vi "GetMeasured.vi"(8 "error in (no error)":errorcluster, 11 "CodeCoverage in":refnum<class "CodeCoverage.lvclass">) -> (0 "error out":errorcluster, 2 "All VIs Measured":path[](array[path]), 3 "CodeCoverage out":refnum<class "CodeCoverage.lvclass">)   [LabVIEW 2019, in "CodeCoverage.lvclass"]
doc: "Returns the paths of all VIs for which code coverage data is available."
uses:
  CodeCoverage.lvclass
  CodeCoverage.lvclass/CodeCoverage.ctl
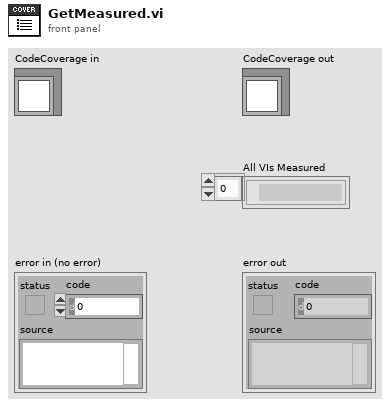
[diagram p1: front panel]
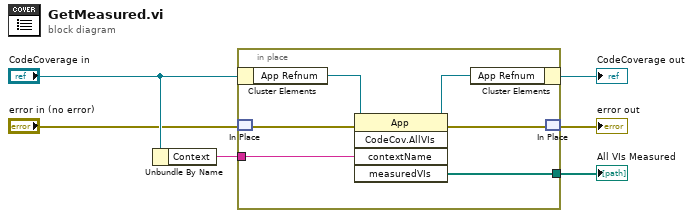
[diagram p0: block diagram]
diagram:
  n1 = Unbundle By Name("CodeCoverage in") -> ("Context"=w6:string)
  n2 = in-place {
    in-place-border: w6 -> [w12]
    in-place-border: [w11] -> w5
    n3 = in-place-cluster #1("CodeCoverage in") -> ("App Refnum"=w10:refnum<vi>)
    n4 = in-place-match #2("error in (no error)") -> (w8:errorcluster)
    n5 = invoke class="App" method="CodeCov.AllVIs"(reference=w10, error in=w8, "contextName"=w12) -> (reference out=w9:refnum<vi>, error out=w7:errorcluster, "measuredVIs"=w11:path[])  [unwired: 2 in, 2 out]
    n6 = in-place-cluster #1("App Refnum"=w9) -> (→"CodeCoverage out":refnum<class "CodeCoverage.lvclass">)
    n7 = in-place-match #2(w7) -> (→"error out":errorcluster)
  }
  "All VIs Measured" <- w5
